vi "Get Type from Class.vi"(3 "Class":string) -> (5 "Channel Type":string)   [LabVIEW 2021, in "CIFChannels.lvclass"]
uses:
  CIFChannels.lvclass
  CIFChannels.lvclass/CIFChannels.ctl
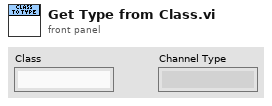
[diagram p1: front panel]
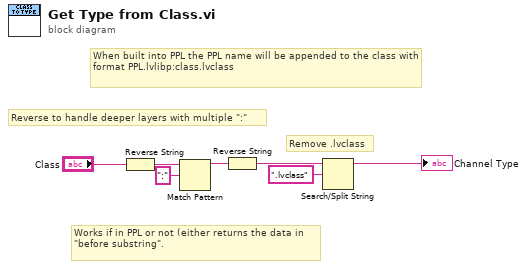
[diagram p0: block diagram]
diagram:
  # "Works if in PPL or not (either returns the data in \"before substring\"."
  # "Remove .lvclass"
  # "Reverse to handle deeper layers with multiple \":\""
  # "When built into PPL the PPL name will be appended to the class with format PPL.lvlibp:class.lvclass"
  n1 = Reverse String(1:"Class") -> (0:w6:string)
  n2 = Match Pattern(string=w6, regular expression=":") -> (before substring=w2:string)  [unwired: 1 in, 3 out]
  n3 = Reverse String(1:w2) -> (0:w3:string)
  n4 = Search/Split String(string=w3, search string/char (-)=".lvclass") -> (substring before match=→"Channel Type":string)  [unwired: 1 in, 2 out]
